vi "Read Transceiver Error.vi"(8 "error in (no error)":errorcluster, 9 "timeout in ms (0)":i32 format="%d ms", 11 "Transceiver Interface in":refnum<class "Transceiver Interface.lvclass">) -> (0 "error out":errorcluster, 1 "empty?":bool, 2 "error":errorcluster, 3 "Transceiver Interface out":refnum<class "Transceiver Interface.lvclass">)   [LabVIEW 2017, in "DSF Core.lvlib" / "Transceiver Interface.lvclass"]
uses:
  Transceiver Interface.lvclass
  C:/Git/DSF/Data Sharing Framework/Source/Core/Engine/Classes/Interfaces/Interface/Interface.lvclass
  Interface/Interface.lvclass/Interface.ctl
  Interface/Get Debug Flags.vi
  Interface/Get Error Queue.vi
  Interface/Errors.vi
  Interface/Error Timeout.vi
  Interface/Read Error Queue.vi
  Interface/Interface.lvclass
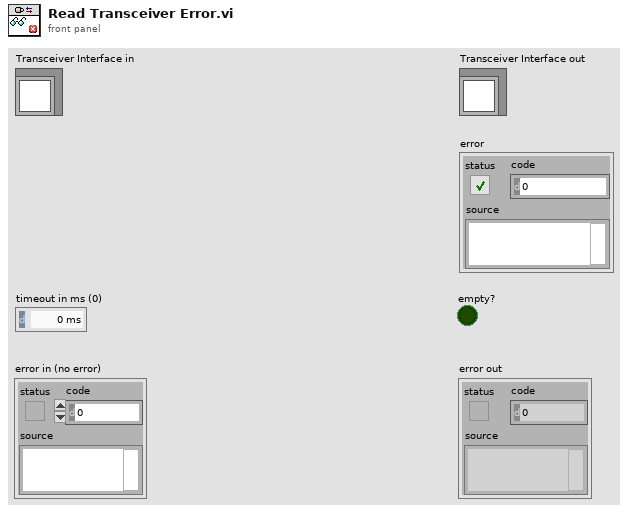
[diagram p1: front panel]
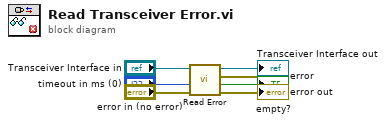
[diagram p0: block diagram]
diagram:
  n1 = call "Read Error.vi"("error in (no error)"="error in (no error)", "timeout in ms (0)"="timeout in ms (0)", "Interface in"="Transceiver Interface in") -> ("error out"=→"error out":errorcluster, "timed out?"=→"empty?":bool, "error"=→"error":errorcluster, "Interface out"=→"Transceiver Interface out":refnum<class "Transceiver Interface.lvclass">)  [unwired: 5 in]
